vi "MultiMFC readNwrite.vi"() -> ()   [LabVIEW 2012]
uses:
  <vilib>/Utility/file.llb/Write To Spreadsheet File (DBL).vi
panel:
  out "odor 2":bool
  out "odor 1":bool
  out "Vol Flow D":dbl
  out "Mass Flow D Chart":dbl(graph)
  out "Mass Flow D":dbl
  out "Set Flow D":dbl
  in  "SetD SCCM\n(200=FullScale)":u16
  out "D Reads":string="D +014.62 +024.78 +0000.0 +0000.0 0000.0     Air\r"
  out "laser power(mW)":dbl
  in  "numSets":dbl=3.0
  in  "numReps":dbl=4.0
  out "VF array":dbl[](array[numeric])=[499.3, 101.3, 18187.0, 1.0, 2.209922211688984]
  out "MF array":dbl[](array[numeric])=[550.0, 100.0, 18187.0, 1.0, 2.209922211688984]
  out "Mass Flow A Chart":dbl(graph)
  out "Vol Flow A":dbl
  out "Mass Flow A":dbl
  out "Set Flow A":dbl
  in  "SetC SCCM\n(200=FullScale)":u16
  out "C Reads":string="C +014.76 +025.18 +0000.0 +0000.0 0000.0     Air\r"
  in  "SetC3 SCCM\n(200=FullScale)":i32=50
  in  "SetC2 SCCM\n(200=FullScale)":i32=50
  in  "SetC1 SCCM\n(200=FullScale)":i32=50
  out "Vol Flow B":dbl
  out "Mass Flow B Chart":dbl(graph)
  out "Mass Flow B":dbl
  out "Set Flow B":dbl
  out "B Reads":string="B +014.77 +025.24 +0000.0 +0000.0 0000.0     Air\r"
  in  "SetB SCCM\n(500=FullScale)":i32
  out "Start Acquisition?":bool
  out "time since start":u32
  out "start time used":u32=1523375771
  out "Vol Flow C":dbl
  out "VF file":path=path "C:/Documents and Settings/Chuntao/Data/090626 test/090626 test VF008.xls"
  out "MF file":path=path "C:/Documents and Settings/Chuntao/Data/090626 test/090626 test MF008.xls"
  out "numStim":u16
  out "old state":bool
  out "base path":path=path "C:/Documents and Settings/Chuntao/Data/090626 test"
  out "base name":string="090626 test"
  out "Stim On?":bool
  in  "Save?":bool
  out "file path":path=path "C:/Documents and Settings/Chuntao/Data/090626 test/090626 test"
  out "Mass Flow C Chart":dbl(graph)
  in  "SetA SCCM\n(2000=FullScale)":i32
  out "Set Flow C":dbl
  out "Mass Flow C":dbl
  out "A Reads":string="A +014.27 +025.36 +00.000 +00.000 00.000     Air\r"
  in  "stop":bool
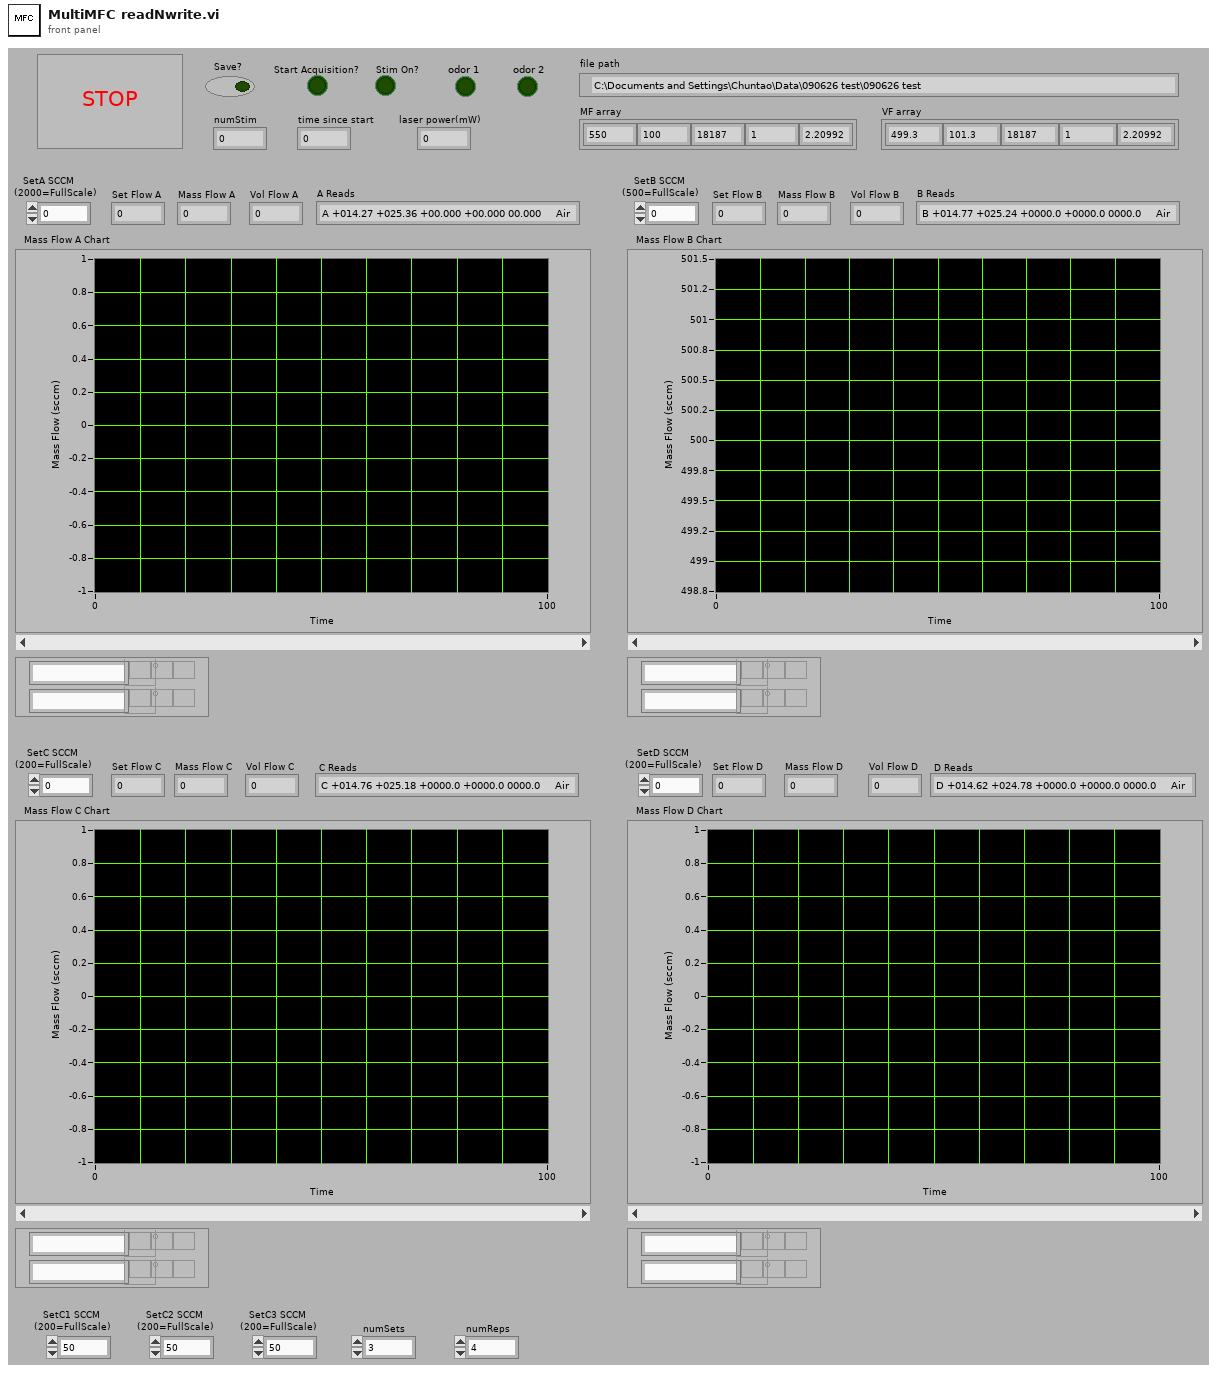
[diagram p1: front panel]
types:
  T1 = cluster{"data[0]":bool, "data[1]":bool, "data[2]":bool}
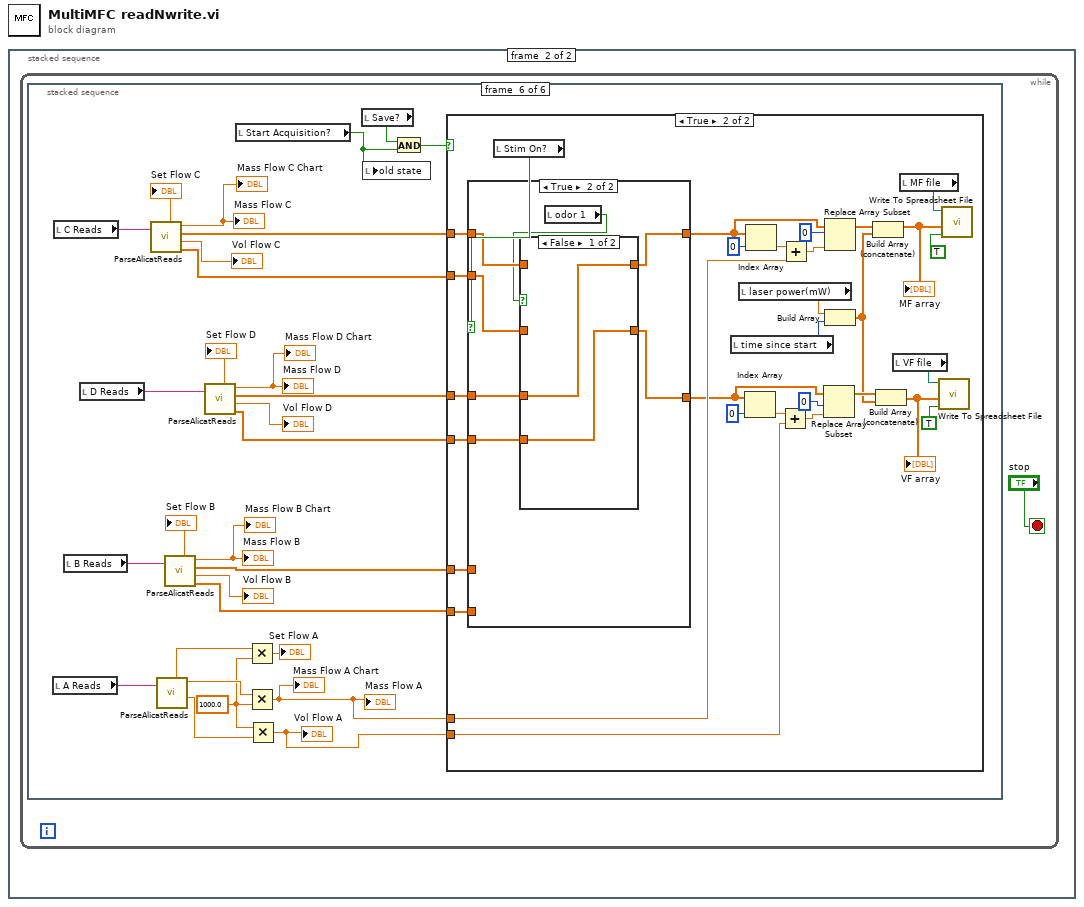
[diagram p0: block diagram]
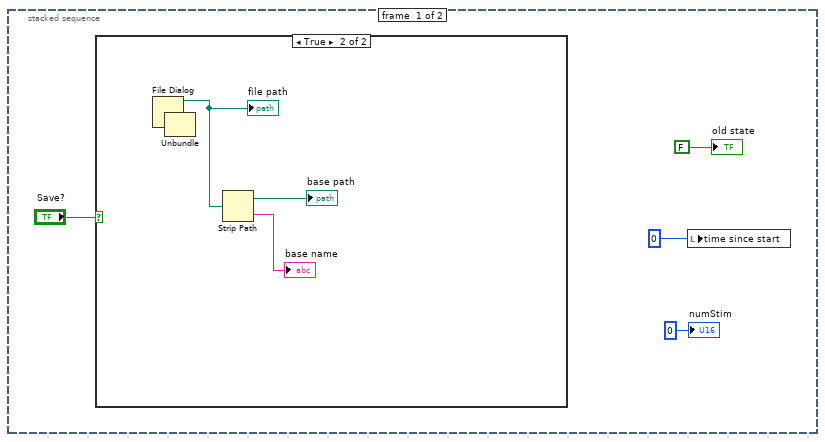
[diagram p2: hidden frame]
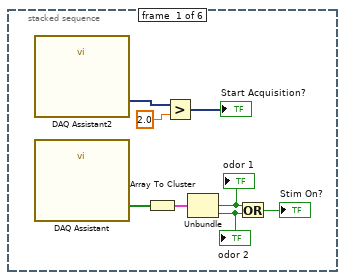
[diagram p4: hidden frame]
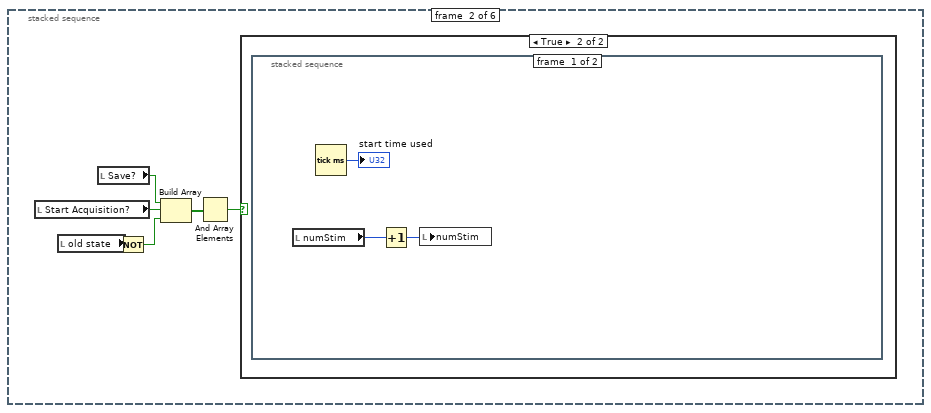
[diagram p5: hidden frame]
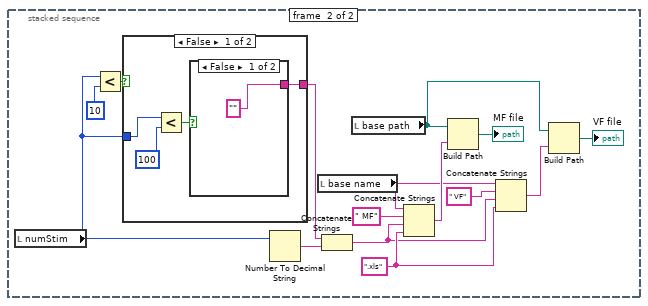
[diagram p7: hidden frame]
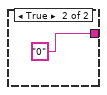
[diagram p8: hidden frame]
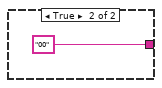
[diagram p9: hidden frame]
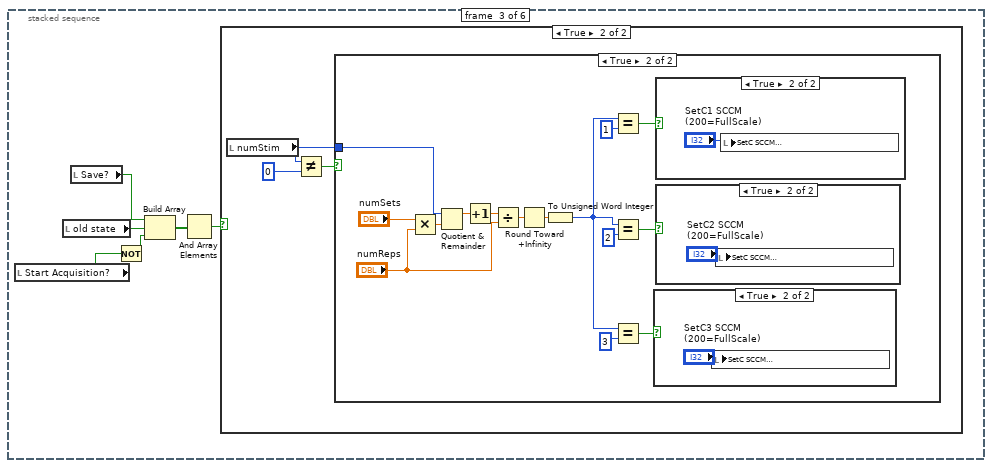
[diagram p10: hidden frame]
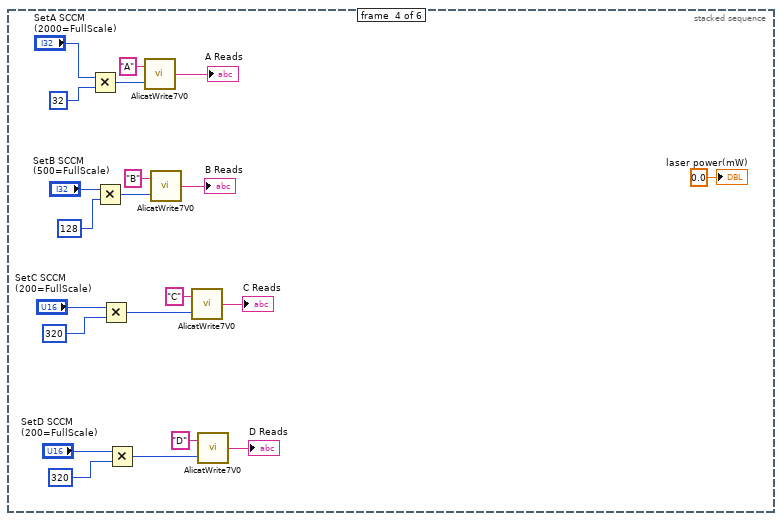
[diagram p16: hidden frame]
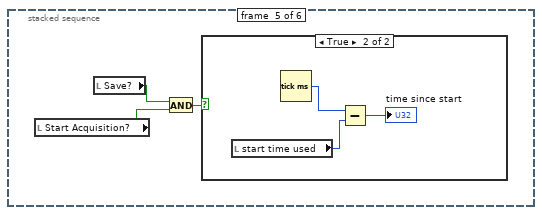
[diagram p17: hidden frame]
diagram:
  n1 = stacked-sequence {
    frame #0 {
      n2 = case shown="True" "Save?" {
        frame False {
        }
        frame True {
          n3 = File Dialog() -> (0:w5:errorcluster, 3:w8:path)  [unwired: 1 in, 8 out]
          "file path" <- w8
          n4 = Unbundle(w5) -> ()  [unwired: 3 out]
          n5 = Strip Path(path=w8) -> (stripped path=→"base path":path, name=→"base name":string)
        }
      }
      n6 = local write "time since start"(u32 0 ("time since stim on")) -> ()
      "old state" <- FALSE ("old state")
      "numStim" <- u16 0 ("numRec")
    }
    frame #1 {
      n7 = while {
        stop <- "stop" stop-if-true
        n8 = stacked-sequence {
          frame #0 {
            n9 = call "DAQ Assistant2"() -> ("data"=w15:dynamicdata)  [unwired: 17 in, 2 out]
            n10 = call "DAQ Assistant"() -> ("data"=w17:bool[])  [unwired: 17 in, 2 out]
            n11 = Array To Cluster(array=w17) -> (cluster=w16:T1)
            n12 = Greater?(x=w15, y=2.0) -> (0:→"Start Acquisition?":dynamicdata)
            n13 = Unbundle(w16) -> ("data[1]"=w12:bool, "data[2]"=w11:bool)  [unwired: 1 out]
            "odor 1" <- w12
            "odor 2" <- w11
            n14 = Or(x=w12, y=w11) -> (x .or. y?=→"Stim On?":bool)
          }
          frame #1 {
            n15 = local read "Start Acquisition?"() -> (w19:bool)
            n16 = local read "old state"() -> (w23:bool)
            n17 = local read "Save?"() -> (w20:bool)
            n18 = Not(x=w23) -> (.not. x?=w18:bool)
            n19 = Build Array(w20, w19, w18) -> (w21:bool[])
            n20 = And Array Elements(Boolean array=w21) -> (logical AND=w22:bool)
            n21 = case shown="True" w22 {
              frame False {
              }
              frame True {
                n22 = stacked-sequence {
                  frame #0 {
                    n23 = local read "numStim"() -> (w26:u16)
                    n24 = Tick Count (ms)() -> (millisecond timer value=→"start time used":u32)
                    n25 = Increment(x=w26) -> (x+1=w25:u16)
                    n26 = local write "numStim"(w25) -> ()
                  }
                  frame #1 {
                    w35 = ".xls" ("string")
                    n27 = local read "numStim"() -> (w27:u16)
                    n28 = Less?(x=w27, y=i16 10) -> (x < y?=w29:bool)
                    n29 = case shown="False" w29 {
                      tunnel: [w42 "00" ("string")] -> w28
                      tunnel: w27 -> [w43 _]
                      frame False {
                        n30 = Less?(x=w43, y=i16 100) -> (x < y?=w45:bool)
                        n31 = case shown="False" w45 {
                          tunnel: ["" ("string") "0" ("string")] -> w42
                          frame False {
                          }
                          frame True {
                          }
                        }
                      }
                      frame True {
                      }
                    }
                    n32 = Number To Decimal String(number=w27) -> (decimal integer string=w31:string)  [unwired: 1 out]
                    n33 = local read "base name"() -> (w37:string)
                    n34 = Concatenate Strings(w28, w31) -> (w32:string)
                    n35 = local read "base path"() -> (w38:path)
                    n36 = Concatenate Strings(w37, " MF" ("string"), w32, w35) -> (w41:string)
                    n37 = Build Path(base path=w38, name or relative path=w41) -> (appended path=→"MF file":path)
                    n38 = Concatenate Strings(w37, " VF" ("string"), w32, w35) -> (w34:string)
                    n39 = Build Path(base path=w38, name or relative path=w34) -> (appended path=→"VF file":path)
                  }
                }
              }
            }
          }
          frame #2 {
            n40 = local read "Start Acquisition?"() -> (w50:bool)
            n41 = local read "old state"() -> (w51:bool)
            n42 = local read "Save?"() -> (w52:bool)
            n43 = Not(x=w50) -> (.not. x?=w49:bool)
            n44 = Build Array(w52, w51, w49) -> (w54:bool[])
            n45 = And Array Elements(Boolean array=w54) -> (logical AND=w53:bool)
            n46 = case shown="True" w53 {
              frame False {
              }
              frame True {
                n47 = local read "numStim"() -> (w56:u16)
                n48 = Not Equal?(x=w56, y=u16 0) -> (x != y?=w57:bool)
                n49 = case shown="True" w57 {
                  tunnel: w56 -> [_ w72]
                  frame False {
                  }
                  frame True {
                    n50 = Multiply(x="numSets", y="numReps") -> (x*y=w60:dbl)
                    n51 = Quotient & Remainder(x=w72, y=w60) -> (x-y*floor(x/y)=w65:dbl)  [unwired: 1 out]
                    n52 = Increment(x=w65) -> (x+1=w59:dbl)
                    n53 = Divide(x=w59, y="numReps") -> (x/y=w64:dbl)
                    n54 = Round Toward +Infinity(x=w64) -> (ceil(x): smallest int >= x=w63:dbl)
                    n55 = To Unsigned Word Integer(number=w63) -> (unsigned 16bit integer=w62:u16)
                    n56 = Equal?(x=w62, y=u16 1) -> (x = y?=w68:bool)
                    n57 = Equal?(x=w62, y=u16 2) -> (x = y?=w67:bool)
                    n58 = Equal?(x=w62, y=u16 3) -> (x = y?=w66:bool)
                    n59 = case shown="True" w66 {
                      frame False {
                      }
                      frame True {
                        n60 = local write "SetC SCCM\n(200=FullScale)"("SetC3 SCCM\n(200=FullScale)") -> ()
                      }
                    }
                    n61 = case shown="True" w68 {
                      frame False {
                      }
                      frame True {
                        n62 = local write "SetC SCCM\n(200=FullScale)"("SetC1 SCCM\n(200=FullScale)") -> ()
                      }
                    }
                    n63 = case shown="True" w67 {
                      frame False {
                      }
                      frame True {
                        n64 = local write "SetC SCCM\n(200=FullScale)"("SetC2 SCCM\n(200=FullScale)") -> ()
                      }
                    }
                  }
                }
              }
            }
          }
          frame #3 {
            n65 = Multiply(x="SetA SCCM\n(2000=FullScale)", y=u16 32) -> (x*y=w94:i32)
            n66 = Multiply(x="SetB SCCM\n(500=FullScale)", y=128) -> (x*y=w89:i32)
            n67 = Multiply(x="SetC SCCM\n(200=FullScale)", y=u16 320) -> (x*y=w81:u16)
            n68 = Multiply(x="SetD SCCM\n(200=FullScale)", y=u16 320) -> (x*y=w76:u16)
            n69 = call "AlicatWrite7V0.vi"("SetPoint\n(64000=FullScale)"=w94, "UnitID"="A") -> ("AlicatResponse"=→"A Reads":string)
            n70 = call "AlicatWrite7V0.vi"("SetPoint\n(64000=FullScale)"=w89, "UnitID"="B") -> ("AlicatResponse"=→"B Reads":string)
            n71 = call "AlicatWrite7V0.vi"("SetPoint\n(64000=FullScale)"=w81, "UnitID"="C") -> ("AlicatResponse"=→"C Reads":string)
            n72 = call "AlicatWrite7V0.vi"("SetPoint\n(64000=FullScale)"=w76, "UnitID"="D") -> ("AlicatResponse"=→"D Reads":string)
            "laser power(mW)" <- 0.0 ("laser power(mW)")
          }
          frame #4 {
            n73 = local read "Start Acquisition?"() -> (w97:bool)
            n74 = local read "Save?"() -> (w98:bool)
            n75 = And(x=w98, y=w97) -> (x .and. y?=w99:bool)
            n76 = case shown="True" w99 {
              frame False {
              }
              frame True {
                n77 = local read "start time used"() -> (w101:u32)
                n78 = Tick Count (ms)() -> (millisecond timer value=w102:u32)
                n79 = Subtract(x=w102, y=w101) -> (x-y=→"time since start":u32)
              }
            }
          }
          frame #5 {
            w111 = 1000.0 ("y")
            n80 = local read "A Reads"() -> (w116:string)
            n81 = local read "C Reads"() -> (w128:string)
            n82 = local read "B Reads"() -> (w127:string)
            n83 = local read "D Reads"() -> (w105:string)
            n84 = call "ParseAlicatReads.vi"("Alicat Reads"=w128) -> ("VF array"=w119:dbl[], "Vol Flow"=→"Vol Flow C":dbl, "MF array"=w120:dbl[], "Mass Flow"=→"Mass Flow C" →"Mass Flow C Chart":dbl, "Set Flow"=→"Set Flow C":dbl)  [unwired: 1 in]
            n85 = call "ParseAlicatReads.vi"("Alicat Reads"=w116) -> ("Vol Flow"=w114:dbl, "Mass Flow"=w115:dbl, "Set Flow"=w112:dbl)  [unwired: 1 in, 2 out]
            n86 = call "ParseAlicatReads.vi"("Alicat Reads"=w127) -> ("VF array"=w117:dbl[], "Vol Flow"=→"Vol Flow B":dbl, "MF array"=w118:dbl[], "Mass Flow"=→"Mass Flow B" →"Mass Flow B Chart":dbl, "Set Flow"=→"Set Flow B":dbl)  [unwired: 1 in]
            n87 = call "ParseAlicatReads.vi"("Alicat Reads"=w105) -> ("VF array"=w103:dbl[], "Vol Flow"=→"Vol Flow D":dbl, "MF array"=w104:dbl[], "Mass Flow"=→"Mass Flow D" →"Mass Flow D Chart":dbl, "Set Flow"=→"Set Flow D":dbl)  [unwired: 1 in]
            n88 = local read "Start Acquisition?"() -> (w129:bool)
            n89 = Multiply(x=w112, y=w111) -> (x*y=→"Set Flow A":dbl)
            n90 = Multiply(x=w115, y=w111) -> (x*y=w110:dbl)
            "Mass Flow A" <- w110
            "Mass Flow A Chart" <- w110
            n91 = Multiply(x=w111, y=w114) -> (x*y=w109:dbl)
            "Vol Flow A" <- w109
            n92 = local read "Save?"() -> (w131:bool)
            n93 = local write "old state"(w129) -> ()
            n94 = And(x=w131, y=w129) -> (x .and. y?=w130:bool)
            n95 = case shown="True" w130 {
              tunnel: w120 -> [_ w156]
              tunnel: w119 -> [_ w155]
              tunnel: w118 -> [_ w154]
              tunnel: w117 -> [_ w153]
              tunnel: w110 -> [_ w150]
              tunnel: w109 -> [_ w142]
              tunnel: w104 -> [_ w133]
              tunnel: w103 -> [_ w132]
              frame False {
              }
              frame True {
                n96 = local read "Stim On?"() -> (w157:bool)
                n97 = case shown="True" w157 {
                  tunnel: w156 -> [_ w170]
                  tunnel: [w163 w169] -> w149
                  tunnel: w155 -> [_ w168]
                  tunnel: [w162 w167] -> w143
                  tunnel: w154 -> [w163 _]
                  tunnel: w153 -> [w162 _]
                  tunnel: w133 -> [_ w166]
                  tunnel: w132 -> [_ w165]
                  frame False {
                  }
                  frame True {
                    n98 = local read "odor 1"() -> (w164:bool)
                    n99 = case shown="False" w164 {
                      tunnel: w170 -> [_ w174]
                      tunnel: [w172 w174] -> w169
                      tunnel: w168 -> [_ w173]
                      tunnel: [w171 w173] -> w167
                      tunnel: w166 -> [w172 _]
                      tunnel: w165 -> [w171 _]
                      frame False {
                      }
                      frame True {
                      }
                    }
                  }
                }
                n100 = local read "time since start"() -> (w135:u32)
                n101 = local read "laser power(mW)"() -> (w136:dbl)
                n102 = Index Array(array=w143, index=0) -> (element=w145:dbl)
                n103 = Index Array(array=w149, index=0) -> (element=w151:dbl)
                n104 = Add(x=w145, y=w142) -> (x+y=w144:dbl)
                n105 = Add(x=w151, y=w150) -> (x+y=w147:dbl)
                n106 = Replace Array Subset(array=w143, new element=w144, index=0) -> (w138:dbl[])
                n107 = Replace Array Subset(array=w149, new element=w147, index=0) -> (w140:dbl[])
                n108 = Build Array(w136, w135) -> (w134:dbl[])
                n109 = Build Array (concatenate)(w140, w134) -> (w139:dbl[])
                "MF array" <- w139
                n110 = Build Array (concatenate)(w138, w134) -> (w137:dbl[])
                "VF array" <- w137
                n111 = local read "VF file"() -> (w158:path)
                n112 = local read "MF file"() -> (w160:path)
                n113 = call-poly <vilib>:"Write To Spreadsheet File.vi"("append to file? (new file:F)"=TRUE, "1D data"=w137, "file path (dialog if empty)"=w158) -> ()  [unwired: 3 in, 3 out]
                n114 = call-poly <vilib>:"Write To Spreadsheet File.vi"("append to file? (new file:F)"=TRUE, "1D data"=w139, "file path (dialog if empty)"=w160) -> ()  [unwired: 3 in, 3 out]
              }
            }
          }
        }
      }
    }
  }
